vi "Settings_Dialog.vi"(8 "error IO 2":errorcluster, 11 "Settings in":T1) -> (0 "error IO":errorcluster, 1 "Cancelled":bool, 3 "Settings out":T1)   [LabVIEW 2022 SP3]
uses:
  controls/Config.ctl
  <vilib>/Utility/xml.llb/Write to XML File(string).vi
panel:
  in  "Homerseklet":dbl=24.0 min=10.0 max=35.0
  in  "Fájl kiválasztása":path
  in  "Cancel Button":bool
  in  "OK Button":bool
  # "°C"
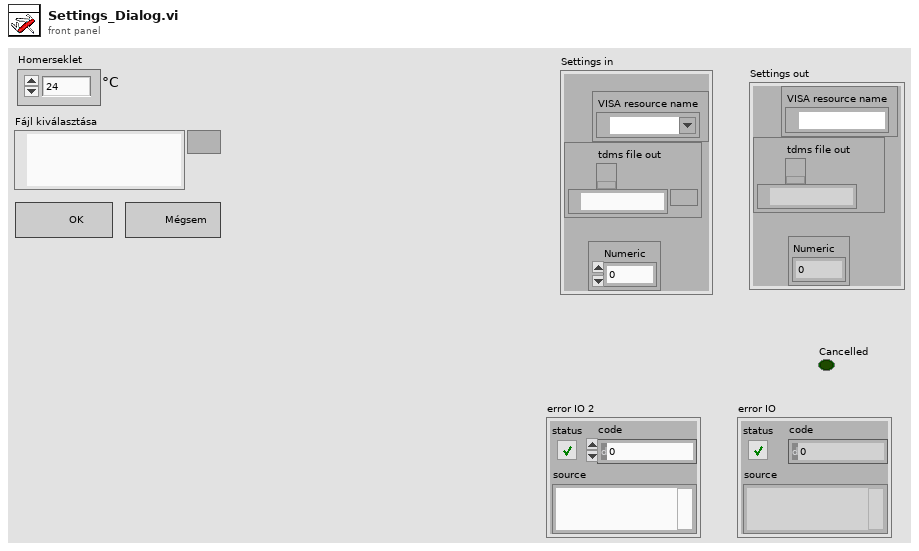
[diagram p1: front panel]
types:
  T1 = typedef "Config.ctl" = cluster{"Hardware":cluster{"VISA resource name":refnum<visa-resource-name>}, "Logging":cluster{"tdms file out":refnum<k34>, "base path":path}, "Set Temp":cluster{"Numeric":dbl}}
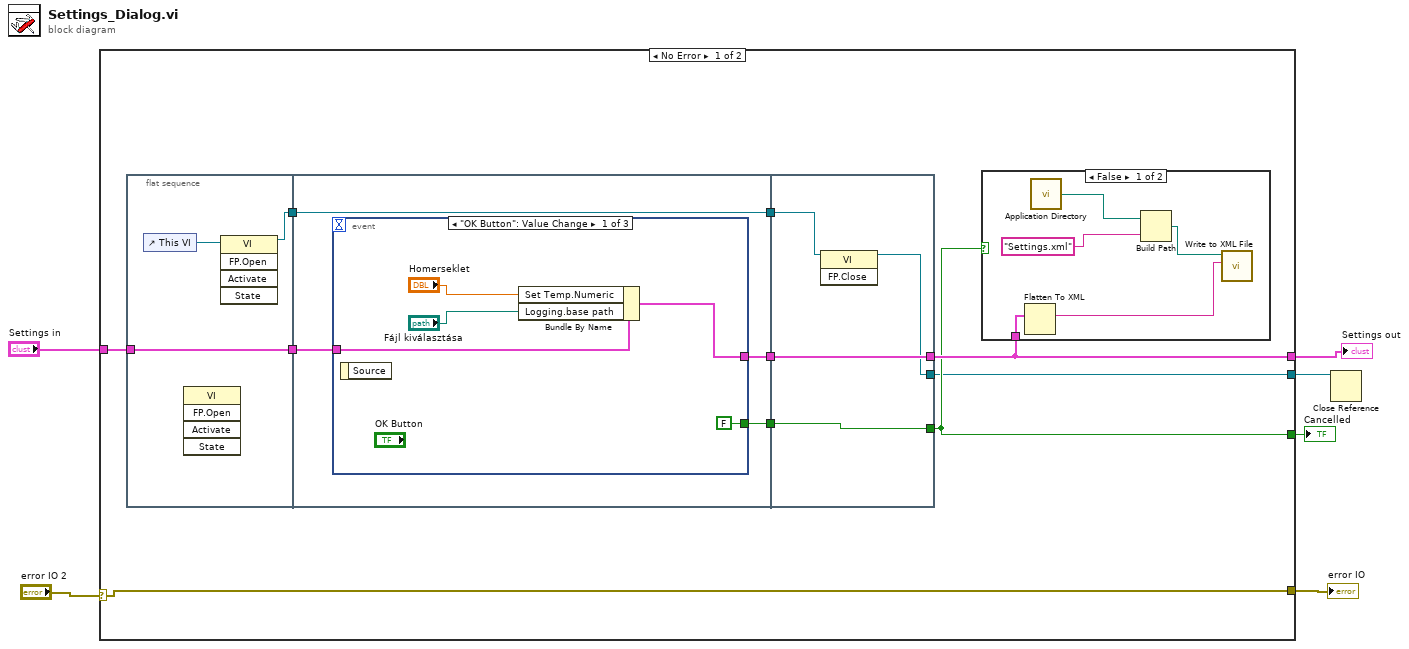
[diagram p0: block diagram]
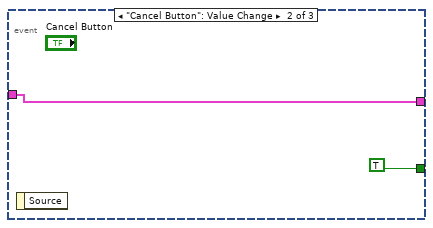
[diagram p3: hidden frame]
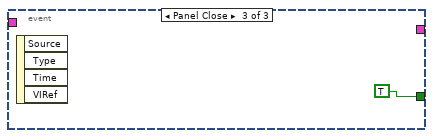
[diagram p4: hidden frame]
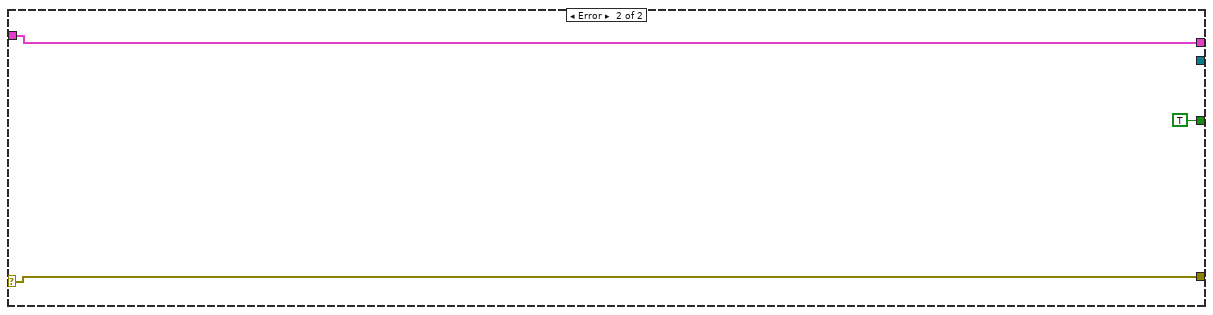
[diagram p5: hidden frame]
diagram:
  n1 = case shown="No Error" "error IO 2" {
    selector: "error IO 2" -> [w10 w42]
    tunnel: "Settings in" -> [w15 w43]
    tunnel: [w12 w43] -> w5
    tunnel: [w11 TRUE] -> w4
    tunnel: [w10 w42] -> w3
    tunnel: [w7 _] -> w1
    frame No Error {
      n2 = flat-sequence {
        tunnel: [w24] -> w16
        tunnel: w15 -> [w24]
        tunnel: [w22] -> w8
        tunnel: w16 -> [w28]
        tunnel: [w27] -> w14
        tunnel: [w26] -> w13
        tunnel: [w25] -> w9
        tunnel: w8 -> [w25]
        tunnel: [w40] -> w12
        tunnel: w14 -> [w40]
        tunnel: [w39] -> w11
        tunnel: w13 -> [w39]
        tunnel: w9 -> [w38]
        tunnel: [w37] -> w7
        frame #0 {
          n3 = control-ref of="This VI"() -> (w23:refnum<vi>)
          n4 = invoke class="VI" method="FP.Open"() -> ()  [unwired: 5 in, 5 out]
          n5 = invoke class="VI" method="FP.Open"(reference=w23) -> (reference out=w22:refnum<vi>)  [unwired: 4 in, 4 out]
        }
        frame #1 {
          n6 = event shown="[0] \"OK Button\": Value Change" {
            selector: _ -> [_ _ _]
            dyn-events: _ -> [_ _ _]
            timeout: _ -> [_ _ _]
            tunnel: w28 -> [w33 w35 _]
            tunnel: [w30 w35 _] -> w27
            tunnel: [FALSE TRUE TRUE] -> w26
            event "OK Button": Value Change {
              n7 = event-data() -> ()  [unwired: 1 in, 1 out]
              n8 = Bundle By Name(cluster=w33, "Set Temp.Numeric"="Homerseklet", "Logging.base path"="Fájl kiválasztása") -> (w30:T1)
            }
            event "Cancel Button": Value Change {
              n9 = event-data() -> ()  [unwired: 1 in, 1 out]
            }
            event Panel Close {
              n10 = event-data() -> ()  [unwired: 1 in, 4 out]
            }
          }
        }
        frame #2 {
          n11 = invoke class="VI" method="FP.Close"(reference=w38) -> (reference out=w37:refnum<vi>)  [unwired: 2 in, 2 out]
        }
      }
      n12 = case shown="False" w11 {
        tunnel: w12 -> [w19 _]
        frame False {
          n13 = Flatten To XML(6:w19) -> (2:w17:string)
          n14 = call <vilib>:"Application Directory.vi"() -> ("Application Directory"=w21:path)
          n15 = Build Path(base path=w21, name or relative path="Settings.xml") -> (appended path=w18:path)
          n16 = call-poly <vilib>:"Write to XML File.vi"("XML Input"=w17, "XML File Path"=w18) -> ()  [unwired: 7 in, 3 out]
        }
        frame True {
        }
      }
    }
    frame Error {
    }
  }
  "Settings out" <- w5
  "Cancelled" <- w4
  "error IO" <- w3
  n17 = Close Reference(reference=w1) -> ()  [unwired: 1 in, 1 out]
